vi "ClusterToIni.vi"() -> ()   [LabVIEW 2018]
uses:
  <vilib>/Utility/config.llb/Write Key (Double).vi
  <vilib>/Utility/config.llb/NI_LVConfig.lvlib
panel:
  in  "configuration file path":path=path "D:/users/Noort/Scan pattern/CreateScanPattern Folder/test.ini"
  in  "Stack":T1={"LED (V)"=1.0, "#z steps"=1, "z step (V)"=1.0, "UV (%)"=0.2} {"UV (%)" format="%#_13g"}
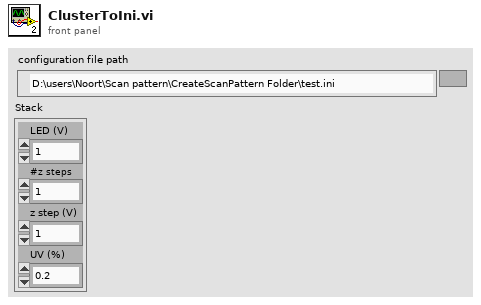
[diagram p1: front panel]
types:
  T1 = cluster{"LED (V)":dbl, "#z steps":i64, "z step (V)":dbl, "UV (%)":dbl}
  T2 = typedef "NI_LVConfig.lvlib/Config Data RefNum.ctl" = refnum<k1>
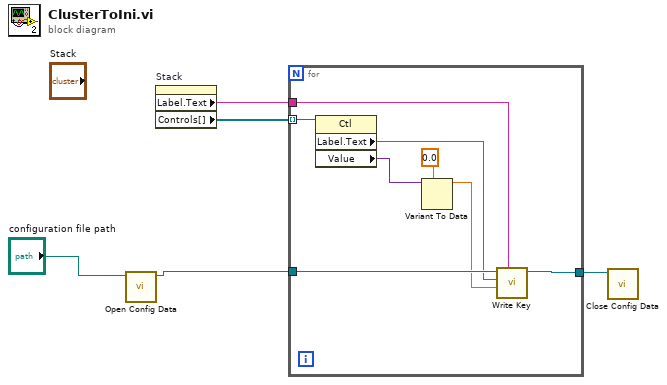
[diagram p0: block diagram]
diagram:
  n1 = call <vilib>:"Open Config Data.vi"("configuration file path"="configuration file path") -> ("refnum"=w3:T2)  [unwired: 8 in, 2 out]
  n2 = property on="Stack" class="Clust (strict)"() -> ("Label.Text"=w2:string, "Controls[]"=w5:refnum<vi>[])  [unwired: 2 in, 2 out]
  n3 = for {
    tunnel: w5 -> [w13] mode=indexing
    tunnel: w3 -> [w12]
    tunnel: w2 -> [w11]
    tunnel: [w6] -> w1
    n4 = property class="Ctl"(reference=w13) -> ("Label.Text"=w10:string, "Value"=w9:variant)  [unwired: 1 in, 2 out]
    n5 = Variant To Data(type=0.0, Variant=w9) -> (data=w8:dbl)  [unwired: 1 in, 1 out]
    n6 = call-poly <vilib>:"Write Key.vi"("section"=w11, "value"=w8, "key"=w10, "refnum"=w12) -> ("refnum out"=w6:T2)  [unwired: 5 in, 2 out]
  }
  n7 = call <vilib>:"Close Config Data.vi"("refnum"=w1) -> ()  [unwired: 9 in, 2 out]
